vi "Begin.vi"(8 "error in":errorcluster) -> (0 "error out":errorcluster)   [LabVIEW 2017]
doc: "Called before other user functions, this VI is expected to open initial I/O refnums, load in file data, and do all program initialization. Notice that the <B>error out</B> terminal is simply used for data flow. Wiring it to other structures or subVIs ensures that this VI runs first."
uses:
  <vilib>/Rock Robotics/SystemInterfaces/DIO/FPGA_DIOPWMChannel.ctl
  <vilib>/Rock Robotics/WPI/Joystick/WPI_JoystickDeviceEnum.ctl
  <vilib>/Rock Robotics/WPI/Solenoid/WPI_SolenoidChannel.ctl
  <vilib>/Rock Robotics/SystemInterfaces/i2clib/i2c_bus.ctl
  <vilib>/Rock Robotics/SystemInterfaces/DIO/FPGA_DIOChannel.ctl
  <vilib>/Rock Robotics/SystemInterfaces/AI/FPGA_AIChannel.ctl
  <userlib>/836-Library/Pneumatics/Support_Code/Pneumatics_Command.ctl
  <userlib>/836-Library/Pneumatics/Support_Code/Pneumatics_Status.ctl
  <vilib>/Rock Robotics/WPI/Solenoid/WPI_SolenoidValue.ctl
  <userlib>/836-Library/Pneumatics/Support_Code/Pneumatics_Position.ctl
  <vilib>/Rock Robotics/WPI/Solenoid/WPI_SolenoidDevRef.ctl
  <vilib>/Rock Robotics/WPI/MotorControl/WPI_MotorControlOpen Talon.vi
  <userlib>/836-Library/Drive/Drive_Code_V2/Drive_Code_Support/DriveTrains/Tank/Tank_4_Motor.vi
  <vilib>/Rock Robotics/WPI/Solenoid/WPI_SolenoidOpenDouble.vi
  <vilib>/Rock Robotics/WPI/Counter/WPI_CounterDigitalInputToDigitalSource.vi
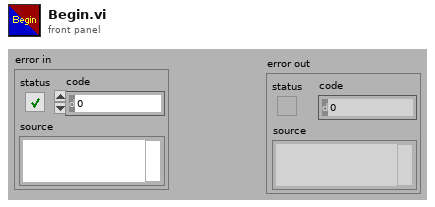
[diagram p1: front panel]
types:
  T1 = typedef "FPGA_AIChannel.ctl" = enum8{"AI 0", "AI 1", "AI 2", "AI 3", "AI MXP 0", "AI MXP 1", "AI MXP 2", "AI MXP 3", "Invalid"}
  T2 = typedef "FPGA_DIOChannel.ctl" = enum8{"DIO 0", "DIO 1", "DIO 2", "DIO 3", "DIO 4", "DIO 5", "DIO 6", "DIO 7", "DIO 8", "DIO 9", "DIO MXP 0", "DIO MXP 1", "DIO MXP 2", "DIO MXP 3", "DIO MXP 4", "DIO MXP 5", "DIO MXP 6", "DIO MXP 7", "DIO MXP 8", "DIO MXP 9", "DIO MXP 10", "DIO MXP 11", "DIO MXP 12", "DIO MXP 13", "DIO MXP 14", "DIO MXP 15", "SPI Port CS1", "SPI Port CS2", "SPI Port CS3", "SPI Port MISO", "SPI Port MOSI", "Invalid"}
  T3 = typedef "i2c_bus.ctl" = enum16{"I2C On-Board", "I2C MXP", "Invalid"}
  T4 = enum8{"ConfigMode", "AccOnly", "MagOnly", "GyroOnly", "AccMag", "AccGyro", "MagGyro", "AMG", "IMU", "Compass", "M4G", "NDOF_FMC_OFF", "NDOF"}
  T5 = typedef "WPI_SolenoidChannel.ctl" = enum8{"Solenoid 0", "Solenoid 1", "Solenoid 2", "Solenoid 3", "Solenoid 4", "Solenoid 5", "Solenoid 6", "Solenoid 7", "Invalid"}
  T6 = typedef "FPGA_DIOPWMChannel.ctl" = enum8{"PWM 0", "PWM 1", "PWM 2", "PWM 3", "PWM 4", "PWM 5", "PWM 6", "PWM 7", "PWM 8", "PWM 9", "PWM MXP 0", "PWM MXP 1", "PWM MXP 2", "PWM MXP 3", "PWM MXP 4", "PWM MXP 5", "PWM MXP 6", "PWM MXP 7", "PWM MXP 8", "PWM MXP 9", "Invalid"}
  T7 = typedef "WPI_JoystickDeviceEnum.ctl" = enum16{"USB 0", "USB 1", "USB 2", "USB 3", "USB 4", "USB 5"}
  T8 = typedef "WPI_SolenoidDevRef.ctl" = cluster{"DevStatus":errorcluster, "Pneumatics Control Module":u8, "Forward Solenoid Channel":T5, "Reverse Solenoid Channel":T5}
  T9 = typedef "WPI_DigitalInputDevRef.ctl" = cluster{"DevStatus":errorcluster, "DIO Channel":T2}
  T10 = typedef "FPGA_CounterEncoderSourceConvertionLVSourceType.ctl" = cluster{"DevStatus":errorcluster, "AnalogTriggerMode?":bool, "DigitalMode":cluster{"DIO Channel":T11}, "AnalogTriggerMode":cluster{"AnalogTriggerIndex":T12, "OutputType":T13}}
  T11 = typedef "FPGA_DIODigitalSourceChannel.ctl" = enum8{"DIO 0", "DIO 1", "DIO 2", "DIO 3", "DIO 4", "DIO 5", "DIO 6", "DIO 7", "DIO 8", "DIO 9", "DIO MXP 0", "DIO MXP 1", "DIO MXP 2", "DIO MXP 3", "DIO MXP 4", "DIO MXP 5", "DIO MXP 6", "DIO MXP 7", "DIO MXP 8", "DIO MXP 9", "DIO MXP 10", "DIO MXP 11", "DIO MXP 12", "DIO MXP 13", "DIO MXP 14", "DIO MXP 15", "Disabled"}
  T12 = typedef "FPGA_AnalogTriggerIndex.ctl" = enum8{"Trig 0", "Trig 1", "Trig 2", "Trig 3", "Trig 4", "Trig 5", "Trig 6", "Trig 7", "Invalid"}
  T13 = typedef "FPGA_AnalogTriggerOutType.ctl" = enum16{"InWindow", "TriggerState", "Rising", "Falling"}
  T14 = typedef "WPI_EncoderDevRef.ctl" = cluster{"DevStatus":errorcluster, "EncoderIndex":T15, "CounterIndex":T16, "DistancePerCount":dbl, "Decoding Type":T17}
  T15 = typedef "FPGA_EncoderIdx.ctl" = enum8{"Enc 0", "Enc 1", "Enc 2", "Enc 3", "Enc 4", "Enc 5", "Enc 6", "Enc 7", "Invalid"}
  T16 = typedef "FPGA_CounterCtrSystemIndex.ctl" = enum8{"Ctr 0", "Ctr 1", "Ctr 2", "Ctr 3", "Ctr 4", "Ctr 5", "Ctr 6", "Ctr 7", "Invalid"}
  T17 = typedef "WPI_EncoderType.ctl" = enum16{"1x", "2x", "4x"}
  T18 = typedef "WPI_AnalogChannelDevRef.ctl" = cluster{"DevStatus":errorcluster, "Analog Channel":T1}
  T19 = typedef "WPI_JoystickDevRef.ctl" = cluster{"Device":T7}
  T20 = typedef "WPI_MotorControlDeviceRef.ctl" = cluster{"DeviceStatus":errorcluster, "Type":T21, "PWM":cluster{"PWM Channel":T6, "DeadBand":T22}, "CAN":cluster{"Device Number":u8, "SetOutput VI Ref":variant, "GetOutput VI Ref":variant, "Enable VI Ref":variant, "Disable VI Ref":variant, "Data":variant}, "Invert":bool, "DIO PWM":cluster{"PWM \"Enable\" Channel":T6, "DIOChannel":T2, "PWM Rate":dbl}}
  T21 = typedef "WPI_MotorControlType.ctl" = enum16{"PWM", "CAN", "DIO PWM"}
  T22 = typedef "WPI_PWMDeadband.ctl" = cluster{"Name":string, "maxPositivePwm":i32, "minPositivePwm":i32, "centerPwm":i32, "maxNegativePwm":i32, "minNegativePwm":i32, "angularRange":u16}
  T23 = typedef "Pneumatics_Notifier.ctl" = cluster{"Command":refnum<notifier>, "Status":refnum<queue>}
  T24 = typedef "Pneumatic_Sensor_Loop.ctl" = cluster{"Status Queue":refnum<queue>, "Status Loop":refnum<k33>, "Relay Value":T25}
  T25 = typedef "WPI_SolenoidValue.ctl" = enum16{"Off", "On", "Forward", "Reverse"}
  T26 = typedef "Solenoid_Control_Loop.ctl" = cluster{"Control Notifier":refnum<notifier>, "Initial Position":T27, "SolenoidDevRef":T8, "Status Loop":refnum<k33>}
  T27 = typedef "Pneumatics_Position.ctl" = enum16{"Forward", "Reverse"}
  T28 = typedef "ImuDevRef.ctl" = cluster{"I2CDevRef":T29, "Valid Cal File?":bool}
  T29 = typedef "WPI_I2CDevRef.ctl" = cluster{"DevStatus":errorcluster, "Device Address":u8, "Handle":i32, "I2C Bus":T3}
  T30 = typedef "Drive_Code_Bundle.ctl" = cluster{"Sensor Data":T31, "RobotDriveDevRef":T33, "Drive Train":T34, "Valid Commands":bool[], "Drive Comand Notifier":refnum<notifier>, "Command Finished?":refnum<k4>, "Command Canceled":refnum<k4>, "PID Inversions":T35, "PID Inputs Notifier":refnum<notifier>, "Cmd Tol Notifier":refnum<notifier>}
  T31 = typedef "Sensor_Cluster.ctl" = cluster{"Gyro Data":cluster{"Gyro RT FIFO":refnum<k33>, "Gyro Current":dbl, "Gyro Hold":dbl}, "Encoder Data":cluster{"Encoder RT FIFO":refnum<k33>, "Encoder Current":dbl, "Encoder Hold":dbl}, "Camera Data":cluster{"Camera RT FIFO":refnum<k33>, "Camera Current":T32}}
  T32 = typedef "Camera_Cluster.ctl" = cluster{" Angle":dbl, "Valid":bool}
  T33 = typedef "WPI_RobotDriveDevRef.ctl" = cluster{"DevStatus":errorcluster, "Motors[]":T20[], "Square Inputs":bool, "Max Output":dbl}
  T34 = typedef "Drive_Trains.ctl" = enum16{"Tank Drive 2 Motor", "Tank Drive 4 Motor", "Tank Drive 6 Motor", "Mecanum Drive", "Kiwi Drive", "Invalid"}
  T35 = typedef "PidInversions.ctl" = cluster{"Distance PID Inverted?":bool, "Yaw PID Inverted?":bool}
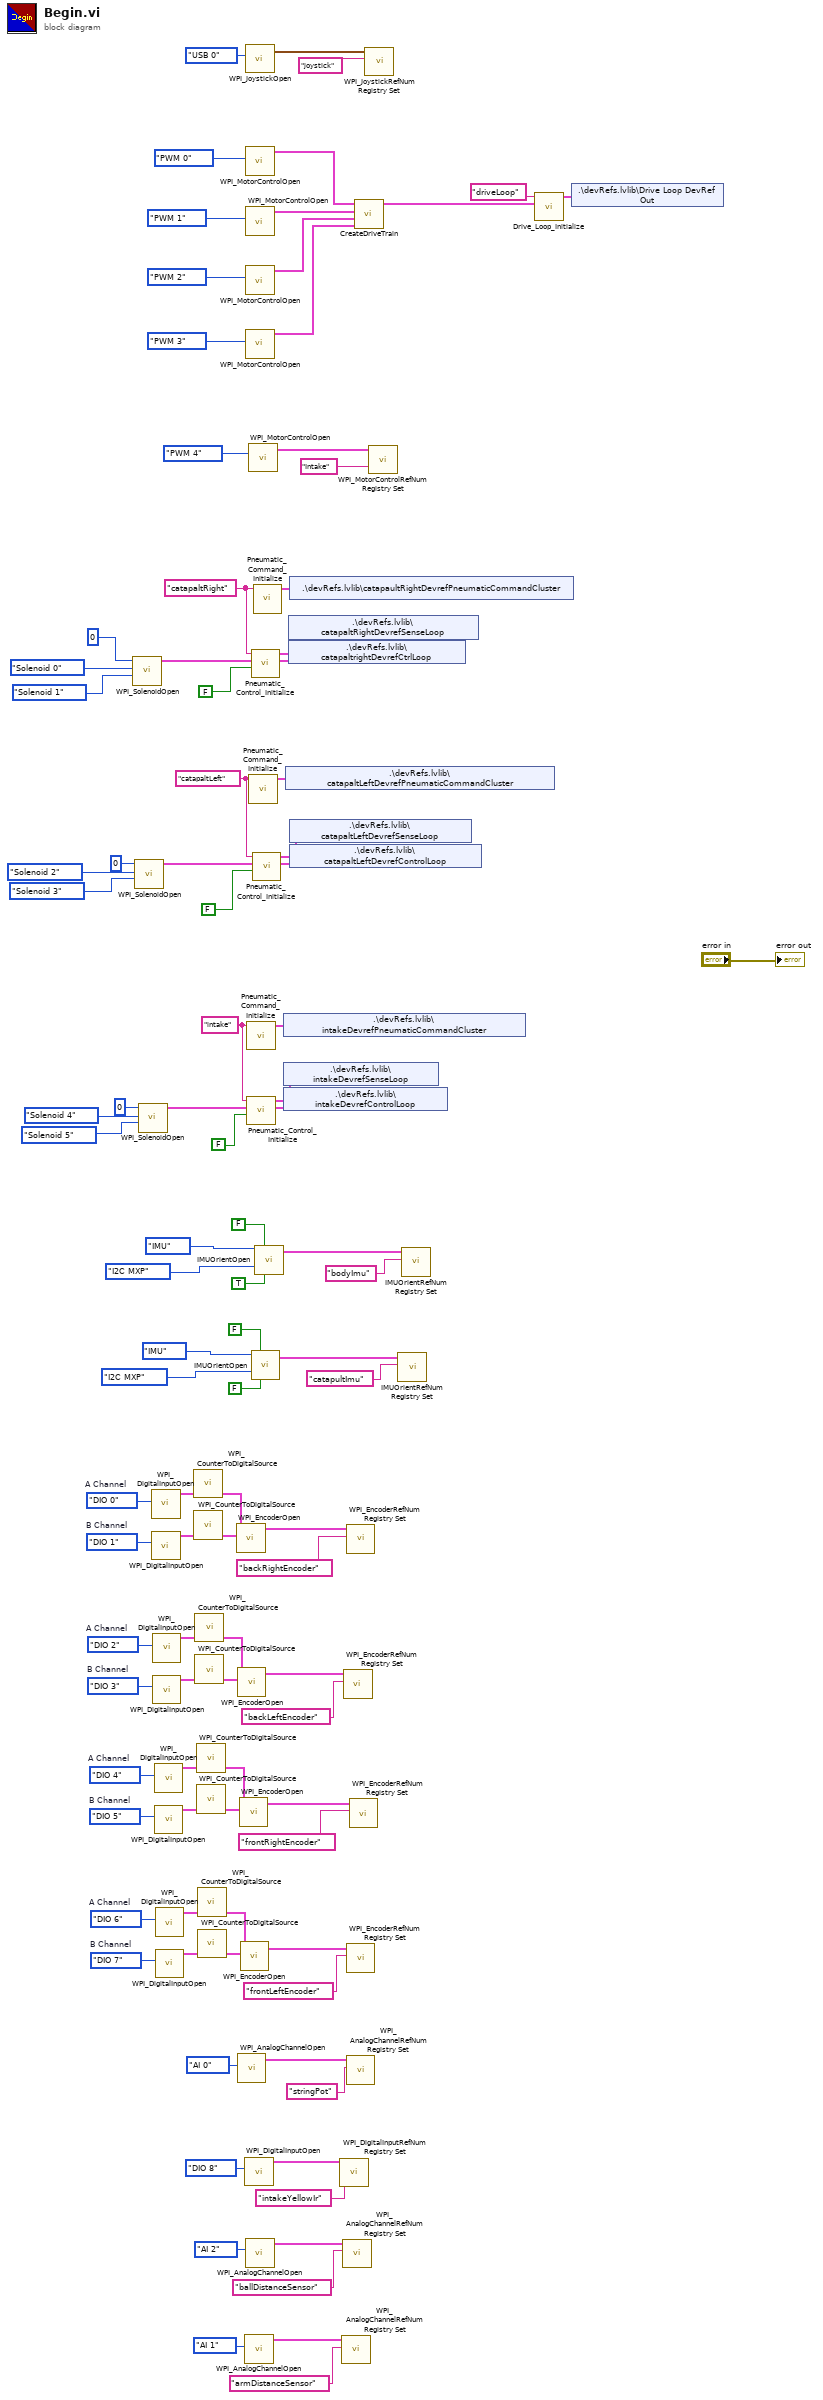
[diagram p0: block diagram]
diagram:
  w24 = FPGA_DIOChannel."DIO 7"  # B Channel
  w23 = FPGA_DIOChannel."DIO 6"  # A Channel
  w13 = FPGA_DIOChannel."DIO 5"  # B Channel
  w14 = FPGA_DIOChannel."DIO 4"  # A Channel
  w33 = FPGA_DIOChannel."DIO 3"  # B Channel
  w34 = FPGA_DIOChannel."DIO 2"  # A Channel
  w44 = FPGA_DIOChannel."DIO 1"  # B Channel
  w43 = FPGA_DIOChannel."DIO 0"  # A Channel
  w80 = "catapaltRight" ("name (unnamed)")
  w79 = "catapaltLeft" ("name (unnamed)")
  w78 = "intake" ("name (unnamed)")
  n1 = call-poly <vilib>:"WPI_SolenoidOpen.vi"("Reverse Solenoid Channel"=WPI_SolenoidChannel."Solenoid 1", "Forward Solenoid Channel"=WPI_SolenoidChannel."Solenoid 0", "Pneumatics Control Module (0)"=u8 0) -> ("SolenoidDevRef"=w83:T8)  [unwired: 7 in, 1 out]
  n2 = call-poly <vilib>:"WPI_SolenoidOpen.vi"("Reverse Solenoid Channel"=WPI_SolenoidChannel."Solenoid 3", "Forward Solenoid Channel"=WPI_SolenoidChannel."Solenoid 2", "Pneumatics Control Module (0)"=u8 0) -> ("SolenoidDevRef"=w82:T8)  [unwired: 7 in, 1 out]
  n3 = call-poly <vilib>:"WPI_SolenoidOpen.vi"("Reverse Solenoid Channel"=WPI_SolenoidChannel."Solenoid 5", "Forward Solenoid Channel"=WPI_SolenoidChannel."Solenoid 4", "Pneumatics Control Module (0)"=u8 0) -> ("SolenoidDevRef"=w81:T8)  [unwired: 7 in, 1 out]
  n4 = call <vilib>:"WPI_DigitalInputOpen.vi"("DIO Channel"=w43) -> ("DigitalInputDevRef"=w40:T9)  [unwired: 1 in, 9 out]
  n5 = call <vilib>:"WPI_DigitalInputOpen.vi"("DIO Channel"=w44) -> ("DigitalInputDevRef"=w41:T9)  [unwired: 1 in, 9 out]
  n6 = call <vilib>:"WPI_DigitalInputOpen.vi"("DIO Channel"=w34) -> ("DigitalInputDevRef"=w37:T9)  [unwired: 1 in, 9 out]
  n7 = call <vilib>:"WPI_DigitalInputOpen.vi"("DIO Channel"=w33) -> ("DigitalInputDevRef"=w36:T9)  [unwired: 1 in, 9 out]
  n8 = call <vilib>:"WPI_DigitalInputOpen.vi"("DIO Channel"=w14) -> ("DigitalInputDevRef"=w17:T9)  [unwired: 1 in, 9 out]
  n9 = call <vilib>:"WPI_DigitalInputOpen.vi"("DIO Channel"=w13) -> ("DigitalInputDevRef"=w16:T9)  [unwired: 1 in, 9 out]
  n10 = call <vilib>:"WPI_DigitalInputOpen.vi"("DIO Channel"=w23) -> ("DigitalInputDevRef"=w20:T9)  [unwired: 1 in, 9 out]
  n11 = call <vilib>:"WPI_DigitalInputOpen.vi"("DIO Channel"=w24) -> ("DigitalInputDevRef"=w21:T9)  [unwired: 1 in, 9 out]
  n12 = call-poly <vilib>:"WPI_CounterToDigitalSource.vi"("DigitalInputDevRef"=w40) -> ("Digital Source"=w39:T10)  [unwired: 6 out]
  n13 = call-poly <vilib>:"WPI_CounterToDigitalSource.vi"("DigitalInputDevRef"=w41) -> ("Digital Source"=w42:T10)  [unwired: 6 out]
  n14 = call-poly <vilib>:"WPI_CounterToDigitalSource.vi"("DigitalInputDevRef"=w37) -> ("Digital Source"=w38:T10)  [unwired: 6 out]
  n15 = call-poly <vilib>:"WPI_CounterToDigitalSource.vi"("DigitalInputDevRef"=w36) -> ("Digital Source"=w35:T10)  [unwired: 6 out]
  n16 = call-poly <vilib>:"WPI_CounterToDigitalSource.vi"("DigitalInputDevRef"=w17) -> ("Digital Source"=w18:T10)  [unwired: 6 out]
  n17 = call-poly <vilib>:"WPI_CounterToDigitalSource.vi"("DigitalInputDevRef"=w16) -> ("Digital Source"=w15:T10)  [unwired: 6 out]
  n18 = call-poly <vilib>:"WPI_CounterToDigitalSource.vi"("DigitalInputDevRef"=w20) -> ("Digital Source"=w19:T10)  [unwired: 6 out]
  n19 = call-poly <vilib>:"WPI_CounterToDigitalSource.vi"("DigitalInputDevRef"=w21) -> ("Digital Source"=w22:T10)  [unwired: 6 out]
  n20 = call <vilib>:"WPI_EncoderOpen.vi"("BSource"=w42, "ASource"=w39) -> ("EncoderDevRef"=w32:T14)  [unwired: 6 in, 3 out]
  n21 = call <vilib>:"WPI_EncoderOpen.vi"("BSource"=w35, "ASource"=w38) -> ("EncoderDevRef"=w31:T14)  [unwired: 6 in, 3 out]
  n22 = call <vilib>:"WPI_AnalogChannelOpen.vi"("Analog Channel"=FPGA_AIChannel."AI 0") -> ("AIDeviceRef"=w11:T18)  [unwired: 9 in, 1 out]
  n23 = call <vilib>:"WPI_EncoderOpen.vi"("BSource"=w15, "ASource"=w18) -> ("EncoderDevRef"=w25:T14)  [unwired: 6 in, 3 out]
  n24 = call <vilib>:"WPI_EncoderOpen.vi"("BSource"=w22, "ASource"=w19) -> ("EncoderDevRef"=w26:T14)  [unwired: 6 in, 3 out]
  n25 = call <vilib>:"WPI_DigitalInputOpen.vi"("DIO Channel"=FPGA_DIOChannel."DIO 8") -> ("DigitalInputDevRef"=w9:T9)  [unwired: 9 in, 1 out]
  n26 = call <vilib>:"WPI_AnalogChannelOpen.vi"("Analog Channel"=FPGA_AIChannel."AI 1") -> ("AIDeviceRef"=w3:T18)  [unwired: 9 in, 1 out]
  n27 = call <vilib>:"WPI_JoystickOpen.vi"("JoystickDevice"=WPI_JoystickDeviceEnum."USB 0") -> ("JoystickDevRef"=w88:T19)  [unwired: 10 in]
  n28 = call-poly <vilib>:"WPI_MotorControlOpen.vi"("PWM Channel"=FPGA_DIOPWMChannel."PWM 0") -> ("MotorControlDeviceRef"=w100:T20)  [unwired: 9 in, 1 out]
  n29 = call-poly <vilib>:"WPI_MotorControlOpen.vi"("PWM Channel"=FPGA_DIOPWMChannel."PWM 1") -> ("MotorControlDeviceRef"=w98:T20)  [unwired: 9 in, 1 out]
  n30 = call-poly <vilib>:"WPI_MotorControlOpen.vi"("PWM Channel"=FPGA_DIOPWMChannel."PWM 2") -> ("MotorControlDeviceRef"=w97:T20)  [unwired: 9 in, 1 out]
  n31 = call-poly <vilib>:"WPI_MotorControlOpen.vi"("PWM Channel"=FPGA_DIOPWMChannel."PWM 3") -> ("MotorControlDeviceRef"=w96:T20)  [unwired: 9 in, 1 out]
  n32 = call <vilib>:"WPI_AnalogChannelOpen.vi"("Analog Channel"=FPGA_AIChannel."AI 2") -> ("AIDeviceRef"=w6:T18)  [unwired: 9 in, 1 out]
  n33 = call <userlib>:"Pneumatic_Command_Initialize.vi"("name (unnamed)"=w78) -> ("Pneumatic Command Cluster"=w59:T23)  [unwired: 9 in, 1 out]
  n34 = call <userlib>:"Pneumatic_Control_Initialize.vi"("Forward?"=FALSE, "SolenoidDevRef"=w81, "name (unnamed)"=w78) -> ("Sense Loop"=w57:T24, "Control Loop"=w58:T26)  [unwired: 7 in]
  n35 = call-poly <vilib>:"WPI_MotorControlOpen.vi"("PWM Channel"=FPGA_DIOPWMChannel."PWM 4") -> ("MotorControlDeviceRef"=w85:T20)  [unwired: 9 in, 1 out]
  n36 = call <userlib>:"Pneumatic_Command_Initialize.vi"("name (unnamed)"=w79) -> ("Pneumatic Command Cluster"=w62:T23)  [unwired: 9 in, 1 out]
  n37 = call <userlib>:"Pneumatic_Control_Initialize.vi"("Forward?"=FALSE, "SolenoidDevRef"=w83, "name (unnamed)"=w80) -> ("Sense Loop"=w63:T24, "Control Loop"=w64:T26)  [unwired: 7 in]
  n38 = call <userlib>:"IMUOrientOpen.vi"("Op Mode"=T4."IMU", "Calibrate?"=FALSE, "I2C Bus"=i2c_bus."I2C MXP", "Alt Adr?"=FALSE) -> ("IMU Dev Ref"=w45:T28)  [unwired: 5 in, 6 out]
  n39 = call <userlib>:"Pneumatic_Control_Initialize.vi"("Forward?"=FALSE, "SolenoidDevRef"=w82, "name (unnamed)"=w79) -> ("Sense Loop"=w60:T24, "Control Loop"=w61:T26)  [unwired: 7 in]
  n40 = call <userlib>:"Pneumatic_Command_Initialize.vi"("name (unnamed)"=w80) -> ("Pneumatic Command Cluster"=w65:T23)  [unwired: 9 in, 1 out]
  n41 = call <userlib>:"IMUOrientOpen.vi"("Op Mode"=T4."IMU", "Calibrate?"=FALSE, "I2C Bus"=i2c_bus."I2C MXP", "Alt Adr?"=TRUE) -> ("IMU Dev Ref"=w56:T28)  [unwired: 5 in, 6 out]
  n42 = shared-variable ".\\devRefs.lvlib\\intakeDevrefPneumaticCommandCluster"(w59) -> ()  [unwired: 1 in, 1 out]
  n43 = shared-variable ".\\devRefs.lvlib\\intakeDevrefSenseLoop"(w57) -> ()  [unwired: 1 in, 1 out]
  n44 = shared-variable ".\\devRefs.lvlib\\intakeDevrefControlLoop"(w58) -> ()  [unwired: 1 in, 1 out]
  n45 = shared-variable ".\\devRefs.lvlib\\catapaltLeftDevrefPneumaticCommandCluster"(w62) -> ()  [unwired: 1 in, 1 out]
  n46 = shared-variable ".\\devRefs.lvlib\\catapaltRightDevrefSenseLoop"(w63) -> ()  [unwired: 1 in, 1 out]
  n47 = shared-variable ".\\devRefs.lvlib\\catapaltrightDevrefCtrlLoop"(w64) -> ()  [unwired: 1 in, 1 out]
  n48 = shared-variable ".\\devRefs.lvlib\\catapaltLeftDevrefSenseLoop"(w60) -> ()  [unwired: 1 in, 1 out]
  n49 = shared-variable ".\\devRefs.lvlib\\catapaltLeftDevrefControlLoop"(w61) -> ()  [unwired: 1 in, 1 out]
  n50 = shared-variable ".\\devRefs.lvlib\\catapaultRightDevrefPneumaticCommandCluster"(w65) -> ()  [unwired: 1 in, 1 out]
  n51 = call <vilib>:"WPI_DigitalInputRefNum Registry Set.vi"("refnum name"="intakeYellowIr", "DigitalInputDevRef"=w9) -> ()  [unwired: 8 in, 2 out]
  n52 = call <vilib>:"WPI_AnalogChannelRefNum Registry Set.vi"("refnum name"="armDistanceSensor", "AIDeviceRef"=w3) -> ()  [unwired: 8 in, 2 out]
  n53 = call <vilib>:"WPI_AnalogChannelRefNum Registry Set.vi"("refnum name"="ballDistanceSensor", "AIDeviceRef"=w6) -> ()  [unwired: 8 in, 2 out]
  n54 = call <vilib>:"WPI_EncoderRefNum Registry Set.vi"("refnum name"="backLeftEncoder", "EncoderDevRef"=w31) -> ()  [unwired: 8 in, 2 out]
  n55 = call <vilib>:"WPI_EncoderRefNum Registry Set.vi"("refnum name"="backRightEncoder", "EncoderDevRef"=w32) -> ()  [unwired: 8 in, 2 out]
  n56 = call <vilib>:"WPI_EncoderRefNum Registry Set.vi"("refnum name"="frontLeftEncoder", "EncoderDevRef"=w26) -> ()  [unwired: 8 in, 2 out]
  n57 = call <vilib>:"WPI_AnalogChannelRefNum Registry Set.vi"("refnum name"="stringPot", "AIDeviceRef"=w11) -> ()  [unwired: 8 in, 2 out]
  n58 = call <vilib>:"WPI_EncoderRefNum Registry Set.vi"("refnum name"="frontRightEncoder", "EncoderDevRef"=w25) -> ()  [unwired: 8 in, 2 out]
  n59 = call-poly <userlib>:"CreateDriveTrain.vi"("Front Right Motor"=w96, "Front Left Motor"=w97, "Rear Right Motor"=w98, "Rear Left Motor"=w100) -> ("DriveClusterOut"=w92:T30)  [unwired: 7 in]
  n60 = call <vilib>:"WPI_JoystickRefNum Registry Set.vi"("refnum name"="joystick", "JoystickDevRef"=w88) -> ()  [unwired: 8 in, 2 out]
  n61 = call <vilib>:"WPI_MotorControlRefNum Registry Set.vi"("refnum name"="Intake", "MotorControlDevRef"=w85) -> ()  [unwired: 8 in, 2 out]
  n62 = call <userlib>:"IMUOrientRefNum Registry Set.vi"("refnum name"="catapultImu", "IMUDevRef in"=w45) -> ()  [unwired: 8 in, 2 out]
  n63 = call <userlib>:"IMUOrientRefNum Registry Set.vi"("refnum name"="bodyImu", "IMUDevRef in"=w56) -> ()  [unwired: 8 in, 2 out]
  n64 = call <userlib>:"Drive_Loop_Initialize.vi"("Drive Train Ref"=w92, "Name"="driveLoop") -> ("Drive DevRef Out"=w90:T30)  [unwired: 9 in]
  n65 = shared-variable ".\\devRefs.lvlib\\Drive Loop DevRef Out"(w90) -> ()  [unwired: 1 in, 1 out]
  "error out" <- "error in"
